vi "average_with_while_loop.vi"() -> ()   [LabVIEW 2019]
panel:
  out "n3":dbl
  out "n2":dbl
  out "n1":dbl
  out "n":dbl
  in  "stop":bool
  out "Ortalama":dbl
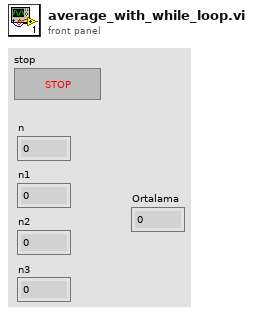
[diagram p1: front panel]
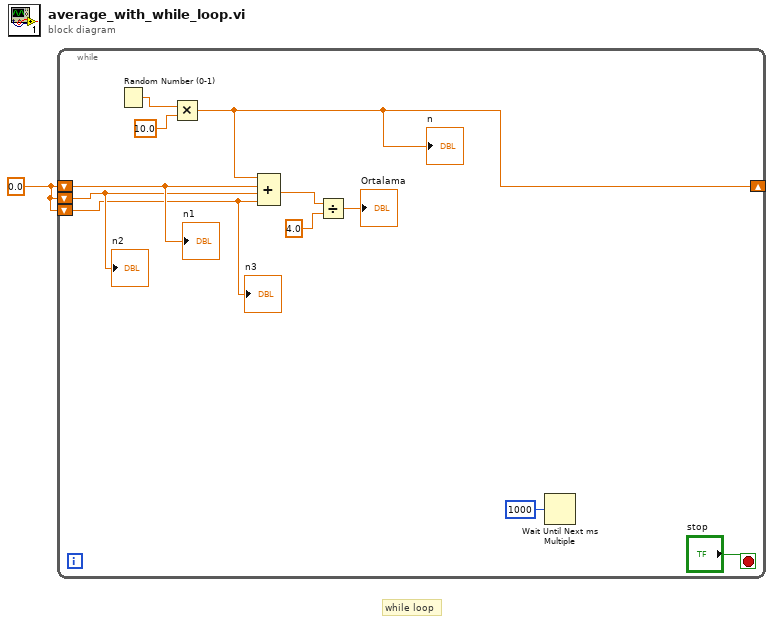
[diagram p0: block diagram]
diagram:
  w1 = 0.0
  # "while loop"
  n1 = while {
    shift-right: [w5] -> _
    shift-left: w1 -> [w4]
    shift-left: w1 -> [w3]
    shift-left: w1 -> [w2]
    stop <- "stop" stop-if-true
    n2 = Random Number (0-1)() -> (number: 0 to 1=w12:dbl)
    n3 = Multiply(x=w12, y=10.0) -> (x*y=w5:dbl)
    "n" <- w5
    n4 = Compound Arithmetic op=ADD(w5, w4, w3, w2) -> (w9:dbl)
    n5 = Divide(x=w9, y=4.0) -> (x/y=→"Ortalama":dbl)
    n6 = Wait Until Next ms Multiple(millisecond multiple=u32 1000) -> ()  [unwired: 1 out]
    "n1" <- w4
    "n2" <- w3
    "n3" <- w2
  }
